vi "Main.vi"() -> ()   [LabVIEW 2020]
uses:
  <vilib>/addons/database/Connection.llb/Conn ObjectReference.ctl
  <vilib>/addons/database/NI_Database_API.lvlib
panel:
  in  "Insert SQL":bool
  in  "Nombre a modificar/eliminar":string
  in  "FechaIngreso":string
  in  "FechaVencimiento":string
  in  "Nombre":string
  in  "Edad":dbl
  out "Result_2D":string[][](array[string])
  in  "Error in":errorcluster
  out "OK Connection":bool
  in  "Stop":bool
  in  "Delete SQL":bool
  in  "Update SQL":bool
  in  "ConnectSQL":bool
  in  "SearchSQL":bool
  # "LabView and SQL\n    Management"
  # "Connection"
  # "Hello World!"
  # "Testing for GitHub"
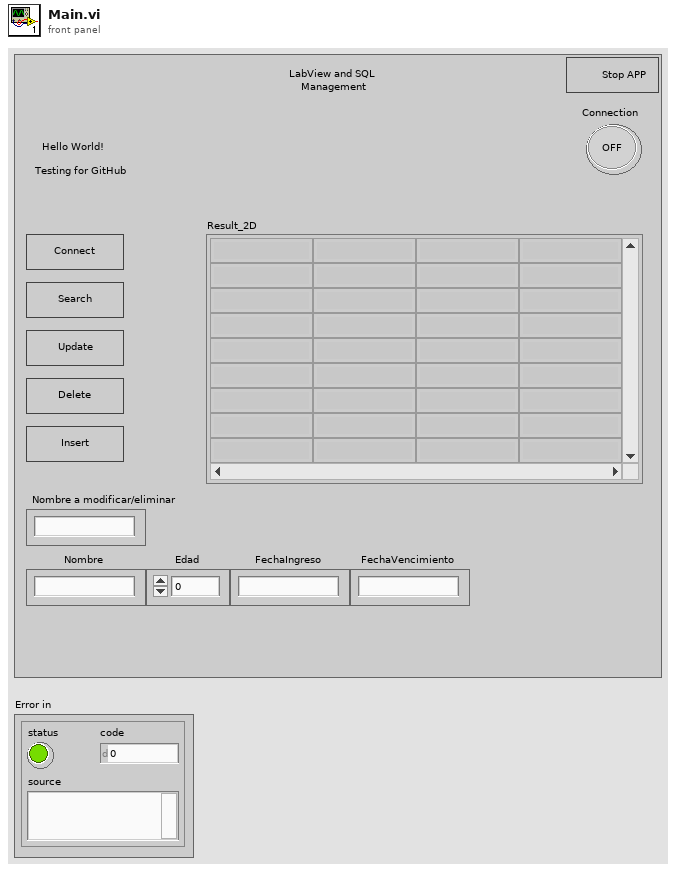
[diagram p1: front panel]
types:
  T1 = cluster{"p1":string, "p2":string, "p3":string, "p4":string, "p5":string, "p6":string, "p7":string, "p8":string, "p9":string, "p10":string}
  T2 = typedef "NI_Database_API.lvlib/Conn ObjectReference.ctl" = refnum<k1>
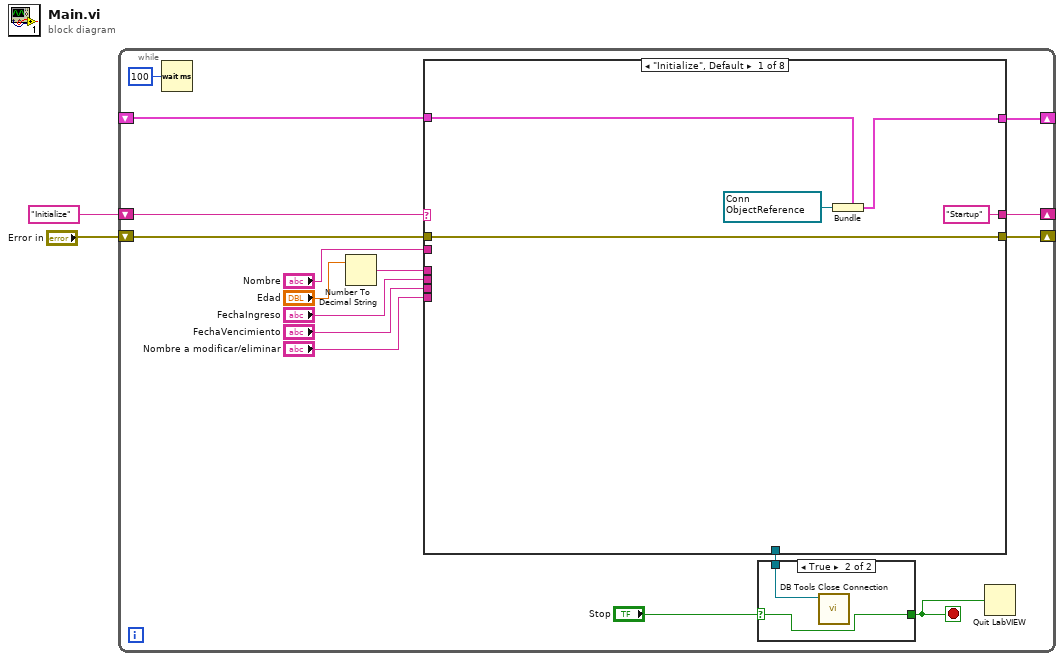
[diagram p0: block diagram]
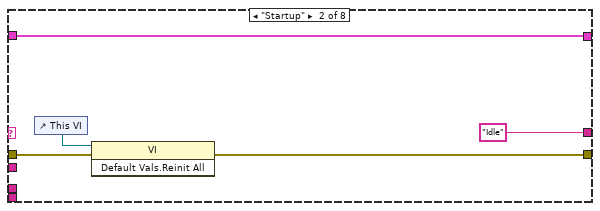
[diagram p3: hidden frame]
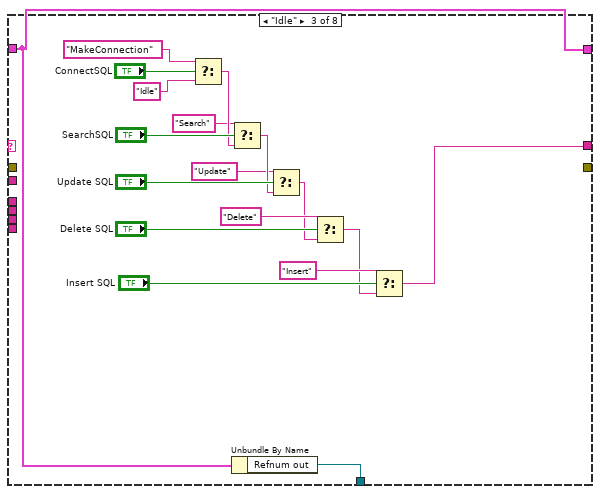
[diagram p4: hidden frame]
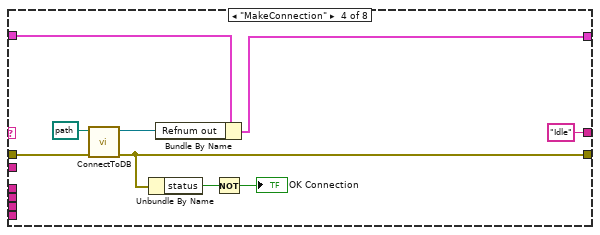
[diagram p5: hidden frame]
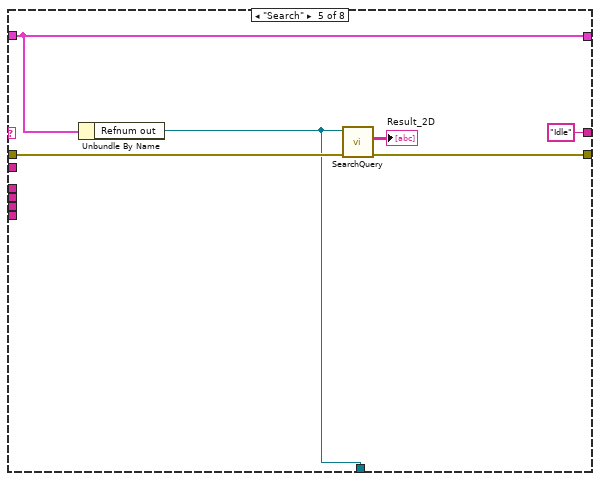
[diagram p6: hidden frame]
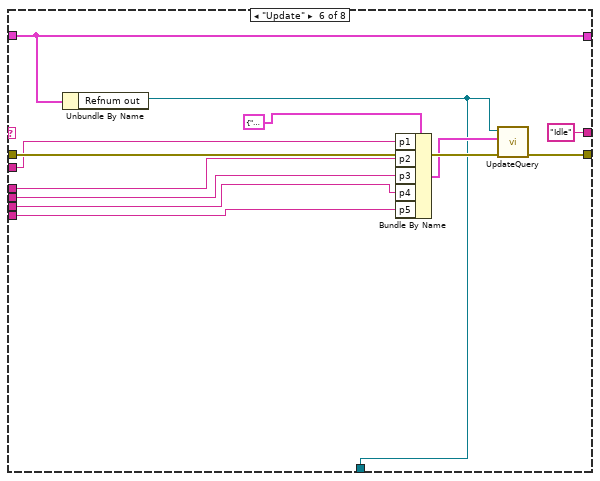
[diagram p7: hidden frame]
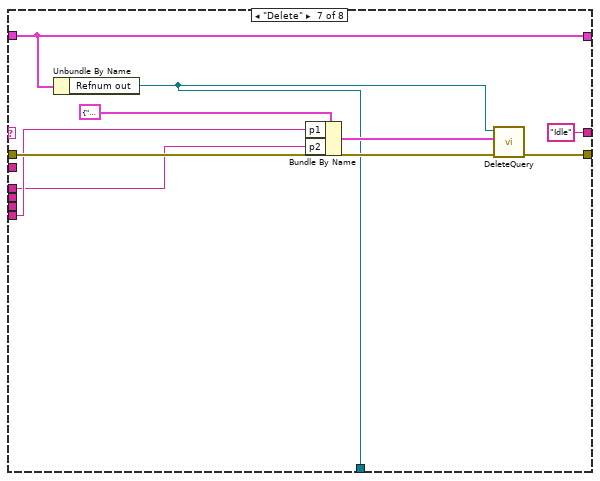
[diagram p8: hidden frame]
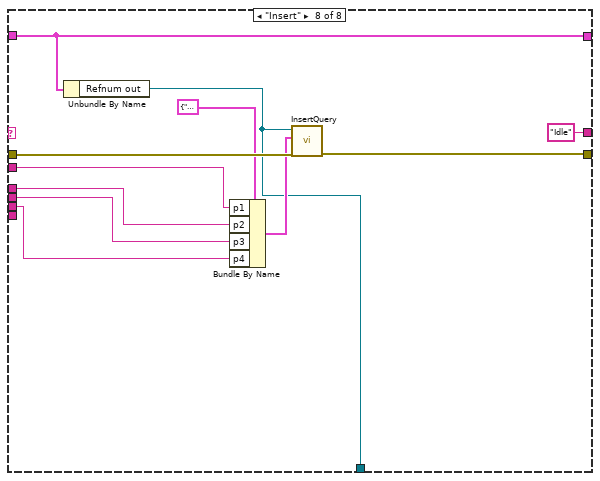
[diagram p9: hidden frame]
diagram:
  n1 = while {
    shift-right: [w15] -> _
    shift-left: "Initialize" -> [w18]
    shift-right: [w16] -> _
    shift-left: "Error in" -> [w17]
    shift-right: [w13] -> _
    shift-left: _ -> [w14]
    stop <- w3 stop-if-true
    n2 = Wait (ms)(milliseconds to wait=u32 100) -> ()  [unwired: 1 out]
    n3 = Number To Decimal String(number="Edad") -> (decimal integer string=w7:string)  [unwired: 1 in]
    n4 = case shown="\"Initialize\", Default" w18 {
      tunnel: w17 -> [w25 w30 _ w57 w62 w75 w84 w95]
      tunnel: [w25 w29 _ w53 w61 w74 w83 w94] -> w16
      tunnel: ["Startup" "Idle" w32 "Idle" "Idle" "Idle" "Idle" "Idle"] -> w15
      tunnel: w14 -> [w23 w27 w38 w56 w63 w72 w82 w93]
      tunnel: [w22 w27 w38 w54 w63 w72 w82 w93] -> w13
      tunnel: [_ _ w37 _ w59 w71 w77 w86] -> w10
      tunnel: "Nombre" -> [_ _ _ _ _ w70 _ w90]
      tunnel: w7 -> [_ _ _ _ _ w69 w78 w89]
      tunnel: "FechaIngreso" -> [_ _ _ _ _ w68 _ w88]
      tunnel: "FechaVencimiento" -> [_ _ _ _ _ w67 _ w87]
      tunnel: "Nombre a modificar/eliminar" -> [_ _ _ _ _ w66 w79 _]
      frame "Initialize", Default {
        w24 = T2 refnum items=["Connection"] ("Refnum out")
        n5 = Bundle(cluster=w23, "Refnum out"=w24) -> (w22:cluster{"Refnum out":T2})
      }
      frame "Startup" {
        n6 = control-ref of="This VI"() -> (w31:refnum<vi>)
        n7 = invoke class="VI" method="Default Vals.Reinit All"(reference=w31, error in=w30) -> (error out=w29:errorcluster)  [unwired: 1 in, 2 out]
      }
      frame "Idle" {
        n8 = Select(t="MakeConnection", s="ConnectSQL", f="Idle") -> (s? t:f=w43:string)
        n9 = Select(t="Search", s="SearchSQL", f=w43) -> (s? t:f=w41:string)
        n10 = Unbundle By Name(w38) -> ("Refnum out"=w37:T2)
        n11 = Select(t="Update", s="Update SQL", f=w41) -> (s? t:f=w34:string)
        n12 = Select(t="Delete", s="Delete SQL", f=w34) -> (s? t:f=w33:string)
        n13 = Select(t="Insert", s="Insert SQL", f=w33) -> (s? t:f=w32:string)
      }
      frame "MakeConnection" {
        n14 = call "ConnectToDB.vi"("Error In"=w57, "UDL_Path"=path "C:/Users/KitKat´s PC/Documents/Maestria/Arquitectura y desarrollo de software/Proyecto_final/Labview/SQL/Cetys-PF_DB.udl") -> ("Error Out"=w53:errorcluster, "Refnum out"=w55:T2)  [unwired: 7 in, 1 out]
        n15 = Unbundle By Name(w53) -> ("status"=w52:bool)
        n16 = Bundle By Name(cluster=w56, "Refnum out"=w55) -> (w54:cluster{"Refnum out":T2})
        n17 = Not(x=w52) -> (.not. x?=→"OK Connection":bool)
      }
      frame "Search" {
        n18 = Unbundle By Name(w63) -> ("Refnum out"=w59:T2)
        n19 = call "SearchQuery.vi"("Error In"=w62, "connection reference"=w59) -> ("Error Out"=w61:errorcluster, "Result_2D"=→"Result_2D":string[][])  [unwired: 5 in, 3 out]
      }
      frame "Update" {
        n20 = Unbundle By Name(w72) -> ("Refnum out"=w71:T2)
        n21 = Bundle By Name(cluster=T1 {"p1"="", "p2"="", "p3"="", "p4"="", "p5"="", "p6"="", "p7"="", "p8"="", "p9"="", "p10"=""} ("input cluster"), "p1"=w70, "p2"=w69, "p3"=w68, "p4"=w67, "p5"=w66) -> (w73:T1)
        n22 = call "UpdateQuery.vi"("Error In"=w75, "input cluster"=w73, "connection reference"=w71) -> ("Error Out"=w74:errorcluster)  [unwired: 4 in, 4 out]
      }
      frame "Delete" {
        n23 = Unbundle By Name(w82) -> ("Refnum out"=w77:T2)
        n24 = Bundle By Name(cluster=T1 {"p1"="", "p2"="", "p3"="", "p4"="", "p5"="", "p6"="", "p7"="", "p8"="", "p9"="", "p10"=""} ("input cluster"), "p1"=w79, "p2"=w78) -> (w80:T1)
        n25 = call "DeleteQuery.vi"("Error In"=w84, "input cluster"=w80, "connection reference"=w77) -> ("Error Out"=w83:errorcluster)  [unwired: 4 in, 4 out]
      }
      frame "Insert" {
        n26 = Unbundle By Name(w93) -> ("Refnum out"=w86:T2)
        n27 = Bundle By Name(cluster=T1 {"p1"="", "p2"="", "p3"="", "p4"="", "p5"="", "p6"="", "p7"="", "p8"="", "p9"="", "p10"=""} ("input cluster"), "p1"=w90, "p2"=w89, "p3"=w88, "p4"=w87) -> (w91:T1)
        n28 = call "InsertQuery.vi"("Error In"=w95, "input cluster"=w91, "connection reference"=w86) -> ("Error Out"=w94:errorcluster)  [unwired: 4 in, 4 out]
      }
    }
    n29 = case shown="True" "Stop" {
      selector: "Stop" -> [w19 w20]
      tunnel: w10 -> [_ w21]
      tunnel: [w19 w20] -> w3
      frame False {
      }
      frame True {
        n30 = call <vilib>:"DB Tools Close Connection.vi"("connection reference"=w21) -> ()  [unwired: 6 in, 1 out]
      }
    }
    n31 = Quit LabVIEW(quit? (T)=w3) -> ()
  }
